vi "Newport Powermeter Control Program(250kHz).vi"() -> ()   [LabVIEW 2018]
panel:
  in  "Wavelength":dbl=830.0
  in  "stop":bool
  in  "Timer(sec)":dbl
  out "Power Meter":cluster{"Power Value":dbl[], "Time":dbl[]}(graph)
  out "Device Name":string
  out "Optical  Power":string[](array[string])
  out "Calibrated Time":dbl=1000.0
  in  "Sample per second":dbl=1.0
  out "Time":dbl[](array[numeric])
  out "Power Value":dbl[](array[numeric])
  # "Real-Time Optical Power Measurement Program"
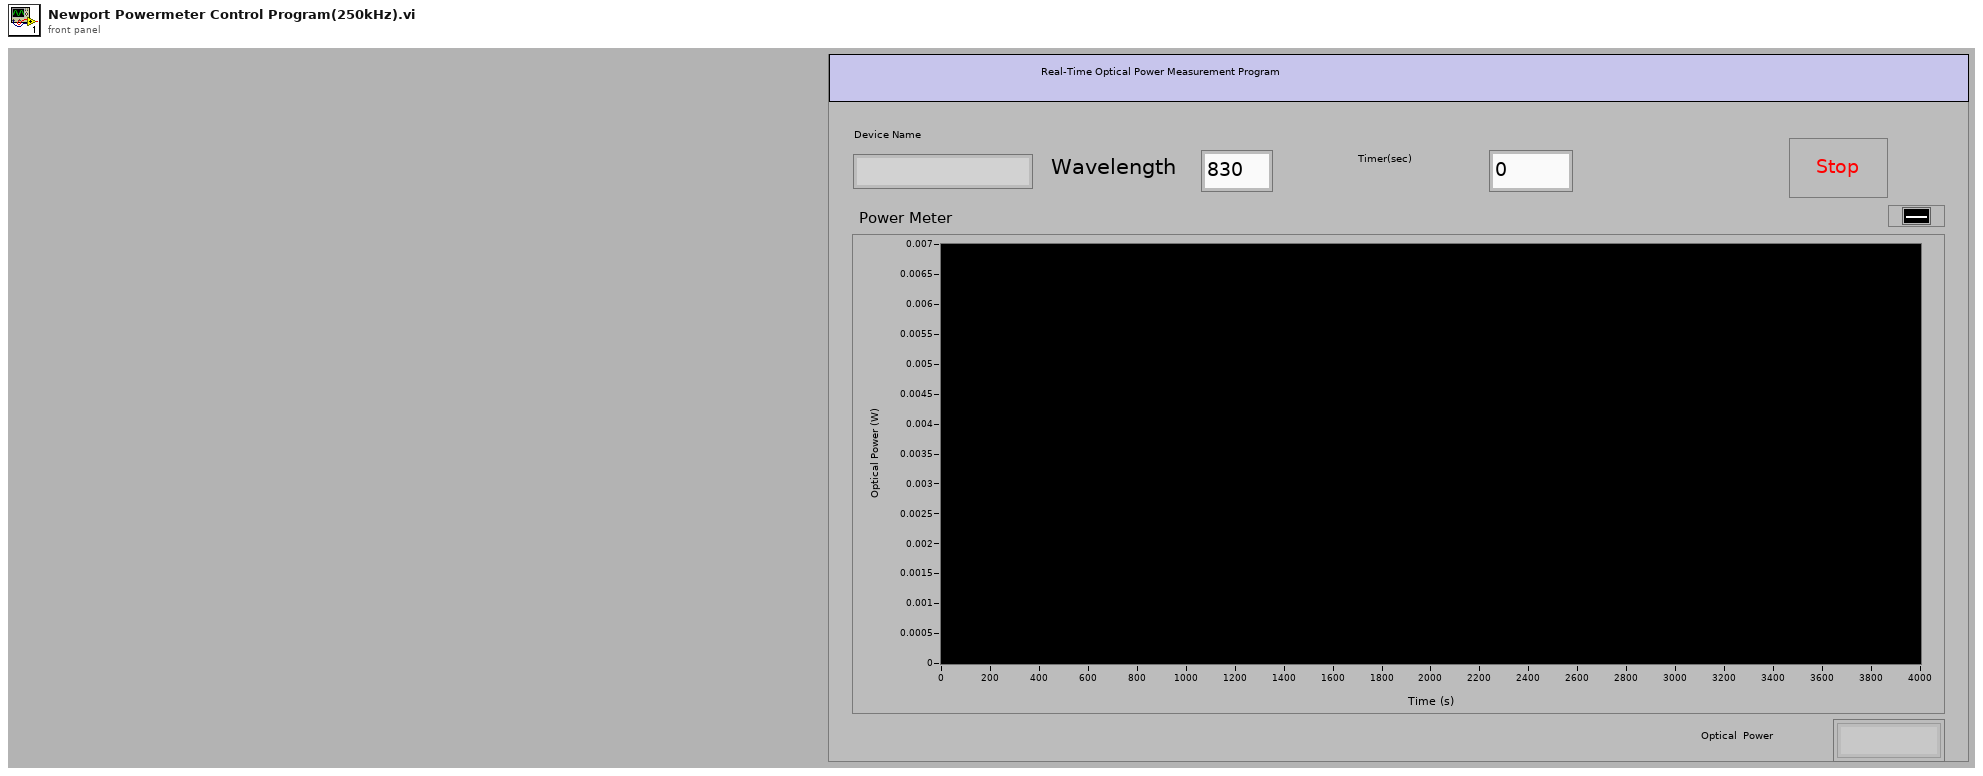
[diagram p1: front panel]
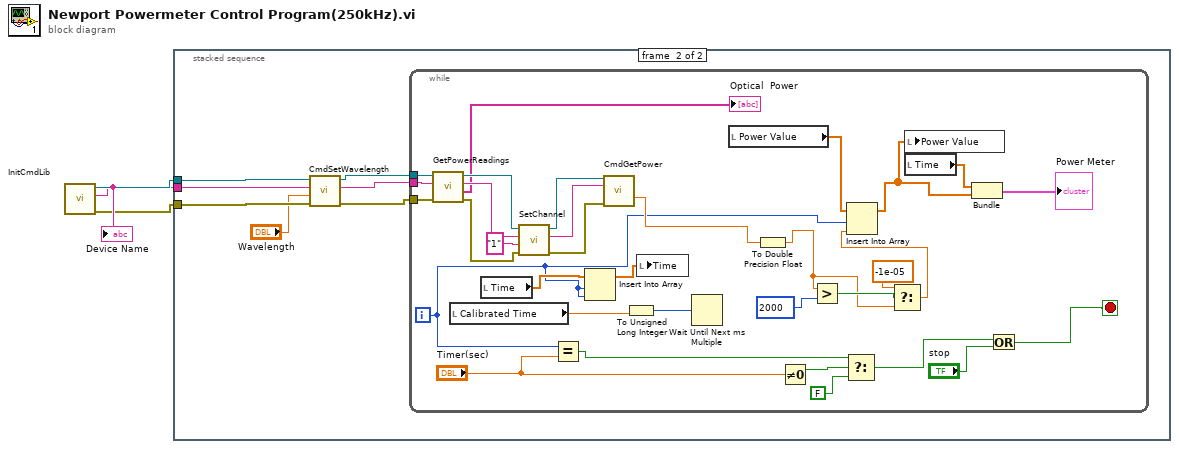
[diagram p0: block diagram]
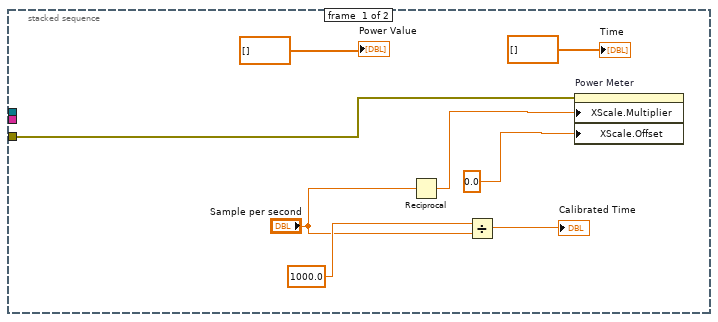
[diagram p2: hidden frame]
diagram:
  n1 = call "InitCmdLib.vi"() -> ("error out"=w1:errorcluster, "Device Key"=w2:string, "CmdLib"=w3:refnum<k24>)  [unwired: 9 in]
  "Device Name" <- w2
  n2 = stacked-sequence {
    tunnel: w3 -> [_ w18]
    tunnel: w2 -> [_ w17]
    tunnel: w1 -> [w4 w16]
    frame #0 {
      n3 = Reciprocal(x="Sample per second") -> (1/x=w6:dbl)
      n4 = Divide(x=1000.0, y="Sample per second") -> (x/y=→"Calibrated Time":dbl)
      n5 = property on="Power Meter" class="XYGraph (엄격한)"(error in=w4, "XScale.Multiplier"=w6, "XScale.Offset"=0.0) -> ()  [unwired: 1 in, 2 out]
      "Power Value" <- dbl[] []
      "Time" <- dbl[] []
    }
    frame #1 {
      n6 = call "CmdSetWavelength.vi"("error in (no error)"=w16, "Wavelength"="Wavelength", "Device Key In"=w17, "CmdLib In"=w18) -> ("error out"=w13:errorcluster, "Device Key Out"=w14:string, "CmdLib Out"=w15:refnum<k24>)  [unwired: 4 in, 1 out]
      n7 = while {
        tunnel: w15 -> [w50]
        tunnel: w14 -> [w49]
        tunnel: w13 -> [w48]
        i -> [w31]
        stop <- w29 stop-if-true
        n8 = call "GetPowerReadings.vi"("error in"=w48, "Device Key In"=w49, "PM Cmds In"=w50) -> ("error out"=w45:errorcluster, "Power Readings"=→"Optical  Power":string[], "Device Key Out"=w46:string, "PM Cmds Out"=w47:refnum<k24>)  [unwired: 1 in]
        n9 = local read "Calibrated Time"() -> (w39:dbl)
        n10 = local read "Time"() -> (w35:dbl[])
        n11 = call "SetChannel.vi"("error in"=w45, "Channel 1 or 2"="1" ("channel"), "Device Key In"=w46, "PM Cmds In"=w47) -> ("error out"=w42:errorcluster, "Device Key Out"=w43:string, "PM Cmds Out"=w44:refnum<k24>)  [unwired: 1 in]
        n12 = Equal?(x=w31, y="Timer(sec)") -> (x = y?=w20:bool)
        n13 = Insert Into Array(array=w35, index=w31, new element=w31) -> (w34:dbl[])
        n14 = call "CmdGetPower.vi"("PM Cmds In"=w44, "Device Key In"=w43, "error in"=w42) -> ("Power Value"=w38:sgl)  [unwired: 8 in, 4 out]
        n15 = To Unsigned Long Integer(number=w39) -> (unsigned 32bit integer=w40:u32)
        n16 = local write "Time"(w34) -> ()
        n17 = Wait Until Next ms Multiple(millisecond multiple=w40) -> ()  [unwired: 1 out]
        n18 = local read "Power Value"() -> (w37:dbl[])
        n19 = To Double Precision Float(number=w38) -> (double precision float=w24:dbl)
        n20 = Not Equal To 0?(x="Timer(sec)") -> (x != 0?=w22:bool)
        n21 = Greater?(x=w24, y=2000) -> (0:w27:bool)
        n22 = Select(t=w20, s=w22, f=FALSE) -> (s? t:f=w21:bool)
        n23 = Select(t=-1e-05, s=w27, f=w24) -> (s? t:f=w25:dbl)
        n24 = Insert Into Array(array=w37, index=w31, new element=w25) -> (w32:dbl[])
        n25 = local write "Power Value"(w32) -> ()
        n26 = local read "Time"() -> (w33:dbl[])
        n27 = Bundle("Time"=w33, "Power Value"=w32) -> (→"Power Meter":cluster{"Time":dbl[], "Power Value":dbl[]})  [unwired: 1 in]
        n28 = Or(x=w21, y="stop") -> (x .or. y?=w29:bool)
      }
    }
  }
